vi "Check Output Status.vi"(0 "CS in":refnum<class "QCS.lvclass">, 1 "I0":T1 {"Current" min=0.0}, 2 "I1":T1 {"Current" min=0.0}, 3 "I2":T1 {"Current" min=0.0}, 4 "I3":T1 {"Current" min=0.0}, 5 "error in (no error)":errorcluster, 6 "Ranges":u8 max=3 format="%08b", 10 "BoardNum":u32, 12 "Force check":bool) -> (14 "CS out":refnum<class "QCS.lvclass">, 15 "I0 out":T1 {"Current" min=0.0}, 16 "I1 out":T1 {"Current" min=0.0}, 17 "I2 out":T1 {"Current" min=0.0}, 18 "I3 out":T1 {"Current" min=0.0}, 19 "error out":errorcluster)   [LabVIEW 2013, in "QCS.lvclass"]
uses:
  Lib.llb/QCS.lvclass
  Lib.llb/CS Data.ctl
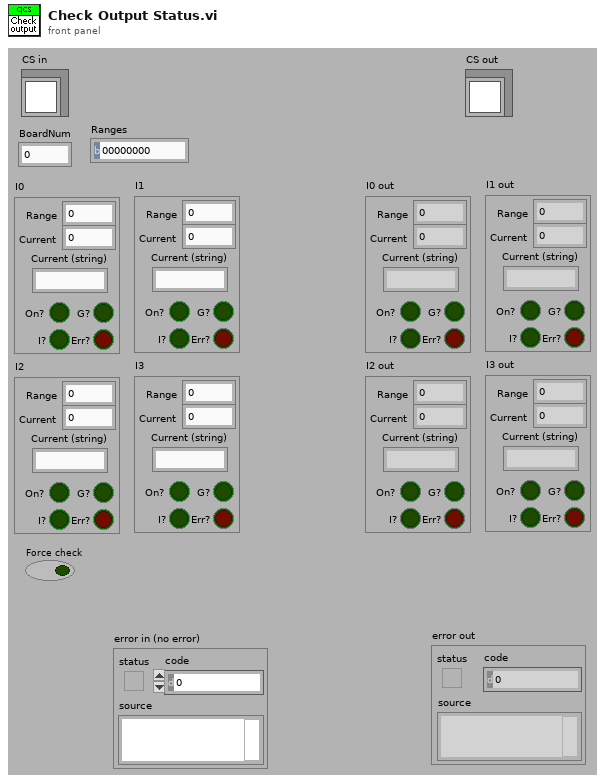
[diagram p1: front panel]
types:
  T1 = typedef "CS Data.ctl" = cluster{"Range":u8, "Current":dbl, "Current (string)":string, "On?":bool, "G?":bool, "I?":bool, "Err?":bool}
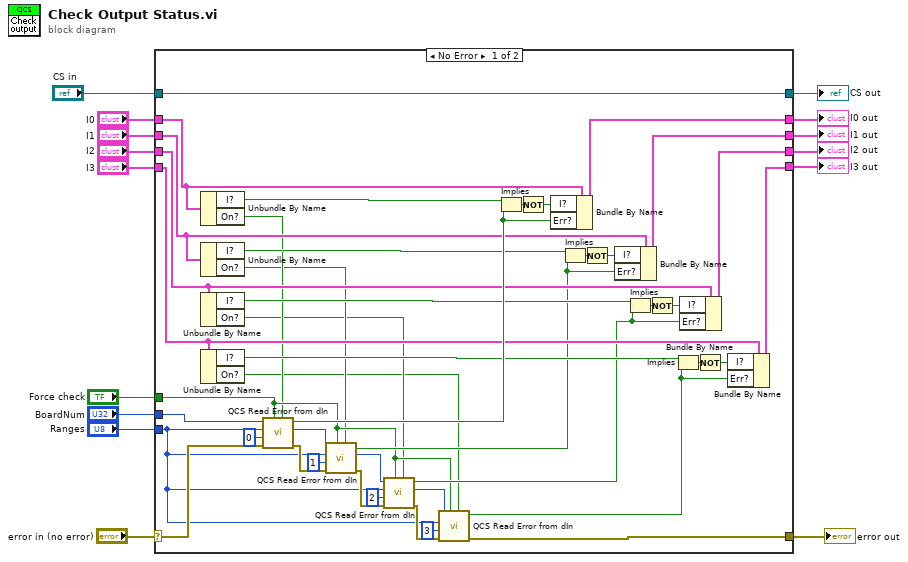
[diagram p0: block diagram]
diagram:
  n1 = case shown="No Error" "error in (no error)" {
    selector: "error in (no error)" -> [w34 w65]
    tunnel: [w24 w65] -> w14
    tunnel: "BoardNum" -> [w59 _]
    tunnel: "Ranges" -> [w23 _]
    tunnel: [w41 w64] -> w10
    tunnel: "I3" -> [w42 w64]
    tunnel: [w45 w63] -> w8
    tunnel: "I2" -> [w46 w63]
    tunnel: [w50 w62] -> w6
    tunnel: "I1" -> [w39 w62]
    tunnel: "I0" -> [w21 w61]
    tunnel: [w58 w61] -> w4
    tunnel: "Force check" -> [w22 _]
    tunnel: "CS in" -> [w16 w60]
    tunnel: [w16 w60] -> w1
    frame No Error {
      n2 = Unbundle By Name(w21) -> ("I?"=w56:bool, "On?"=w20:bool)
      n3 = Unbundle By Name(w39) -> ("I?"=w52:bool, "On?"=w19:bool)
      n4 = Unbundle By Name(w46) -> ("I?"=w48:bool, "On?"=w18:bool)
      n5 = Unbundle By Name(w42) -> ("I?"=w43:bool, "On?"=w17:bool)
      n6 = call "QCS Read Error from dIn.vi"("Current on?"=w20, "Force check"=w22, "error IO"=w34, "Channel"=u8 0, "Ranges"=w23, "BoardNum"=w59) -> ("error out"=w36:errorcluster, "BoardNum out"=w35:u32, "Error?"=w55:bool)  [unwired: 1 in]
      n7 = call "QCS Read Error from dIn.vi"("Current on?"=w19, "Force check"=w22, "error IO"=w36, "Channel"=u8 1, "Ranges"=w23, "BoardNum"=w35) -> ("error out"=w31:errorcluster, "BoardNum out"=w32:u32, "Error?"=w33:bool)  [unwired: 1 in]
      n8 = call "QCS Read Error from dIn.vi"("Current on?"=w18, "Force check"=w22, "error IO"=w31, "Channel"=u8 2, "Ranges"=w23, "BoardNum"=w32) -> ("error out"=w26:errorcluster, "BoardNum out"=w27:u32, "Error?"=w29:bool)  [unwired: 1 in]
      n9 = call "QCS Read Error from dIn.vi"("Current on?"=w17, "Force check"=w22, "error IO"=w26, "Channel"=u8 3, "Ranges"=w23, "BoardNum"=w27) -> ("error out"=w24:errorcluster, "Error?"=w25:bool)  [unwired: 1 in, 1 out]
      n10 = Implies(1:w55, 2:w56) -> (0:w57:bool)
      n11 = Not(x=w57) -> (.not. x?=w54:bool)
      n12 = Bundle By Name(cluster=w21, "I?"=w54, "Err?"=w55) -> (w58:T1)
      n13 = Implies(1:w33, 2:w52) -> (0:w51:bool)
      n14 = Not(x=w51) -> (.not. x?=w53:bool)
      n15 = Bundle By Name(cluster=w39, "I?"=w53, "Err?"=w33) -> (w50:T1)
      n16 = Implies(1:w29, 2:w48) -> (0:w49:bool)
      n17 = Not(x=w49) -> (.not. x?=w47:bool)
      n18 = Implies(1:w25, 2:w43) -> (0:w40:bool)
      n19 = Bundle By Name(cluster=w46, "I?"=w47, "Err?"=w29) -> (w45:T1)
      n20 = Not(x=w40) -> (.not. x?=w44:bool)
      n21 = Bundle By Name(cluster=w42, "I?"=w44, "Err?"=w25) -> (w41:T1)
    }
    frame Error {
    }
  }
  "error out" <- w14
  "I1 out" <- w6
  "I3 out" <- w10
  "I2 out" <- w8
  "I0 out" <- w4
  "CS out" <- w1
